vi "船舶健康监测7.22.vi"() -> ()   [LabVIEW 2018]
uses:
  D:/labview2018/LabVIEW 2018/examples/Connectivity/Python/support/PythonVersionsEnum.ctl
  <vilib>/Instr/_visa.llb/VISA Configure Serial Port (Instr).vi
  <vilib>/picture/3D Picture Control/Object/Add Object (no reference).vi
  <vilib>/picture/3D Picture Control/NI_3D Picture Control.lvlib
panel:
  in  "钉钉机器人开关":bool
  in  "Python版本":T1
  in  "VISA资源名称":refnum<visa-resource-name>
  out "?":refnum<vi>(3d-picture)
  out "?":refnum<vi>(3d-picture)
  out "?":refnum<vi>(3d-picture)
  out "?":i32(graph)
  out "?":i32(graph)
  out "?":i32(graph)
  out "?":i32(graph)
  out "?":i32(graph)
  in  "baud rate (9600)":u32=9600 caption="波特率"
  out "?":i32(graph)
  out "?":string
  out "下弯超过阈值":bool
  out "上弯超过阈值":bool
  out "原始数据":string
  in  "下阈值":dbl
  in  "上阈值":dbl
  in  "?":bool
  # "船舶健康监测数据显示平台"
  # "功能与使用说明：\n1.应变：实现实时图标显示应变值；阈值报警；周期内统计上传至onenet平台；钉钉机器人报警系统；保存至.txt格式文件。\n\n2.温湿度：实现实时图表显示；保存至.txt文件；\n\n3.姿态：实现实时图表显示；三维动态显示"
  # "应变"
  # "温度"
  # "Roll"
  # "湿度"
  # "Pitch"
  # "阈值\n报警"
  # "钉钉\n机器人"
  # "未开发"
  # "写入\n文件\n.txt"
  # "串口配置"
  # "Yallh"
  # "未开发"
  # "未开发"
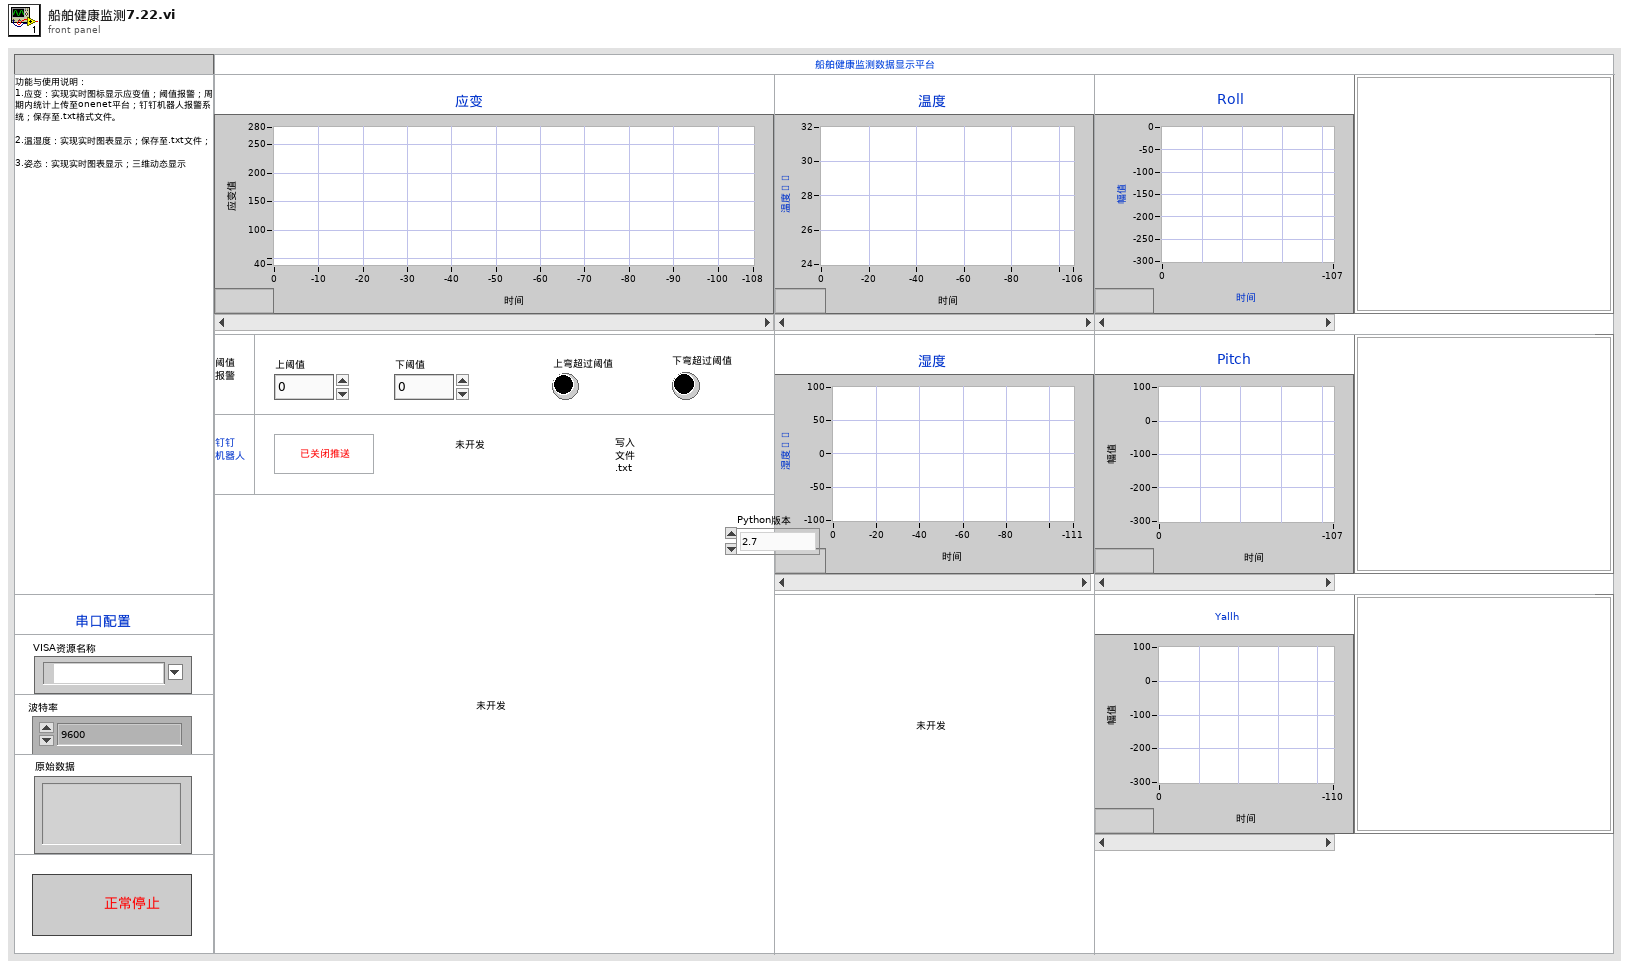
[diagram p1: front panel]
types:
  T1 = typedef "PythonVersionsEnum.ctl" = enum16{"2.7", "3.6"}
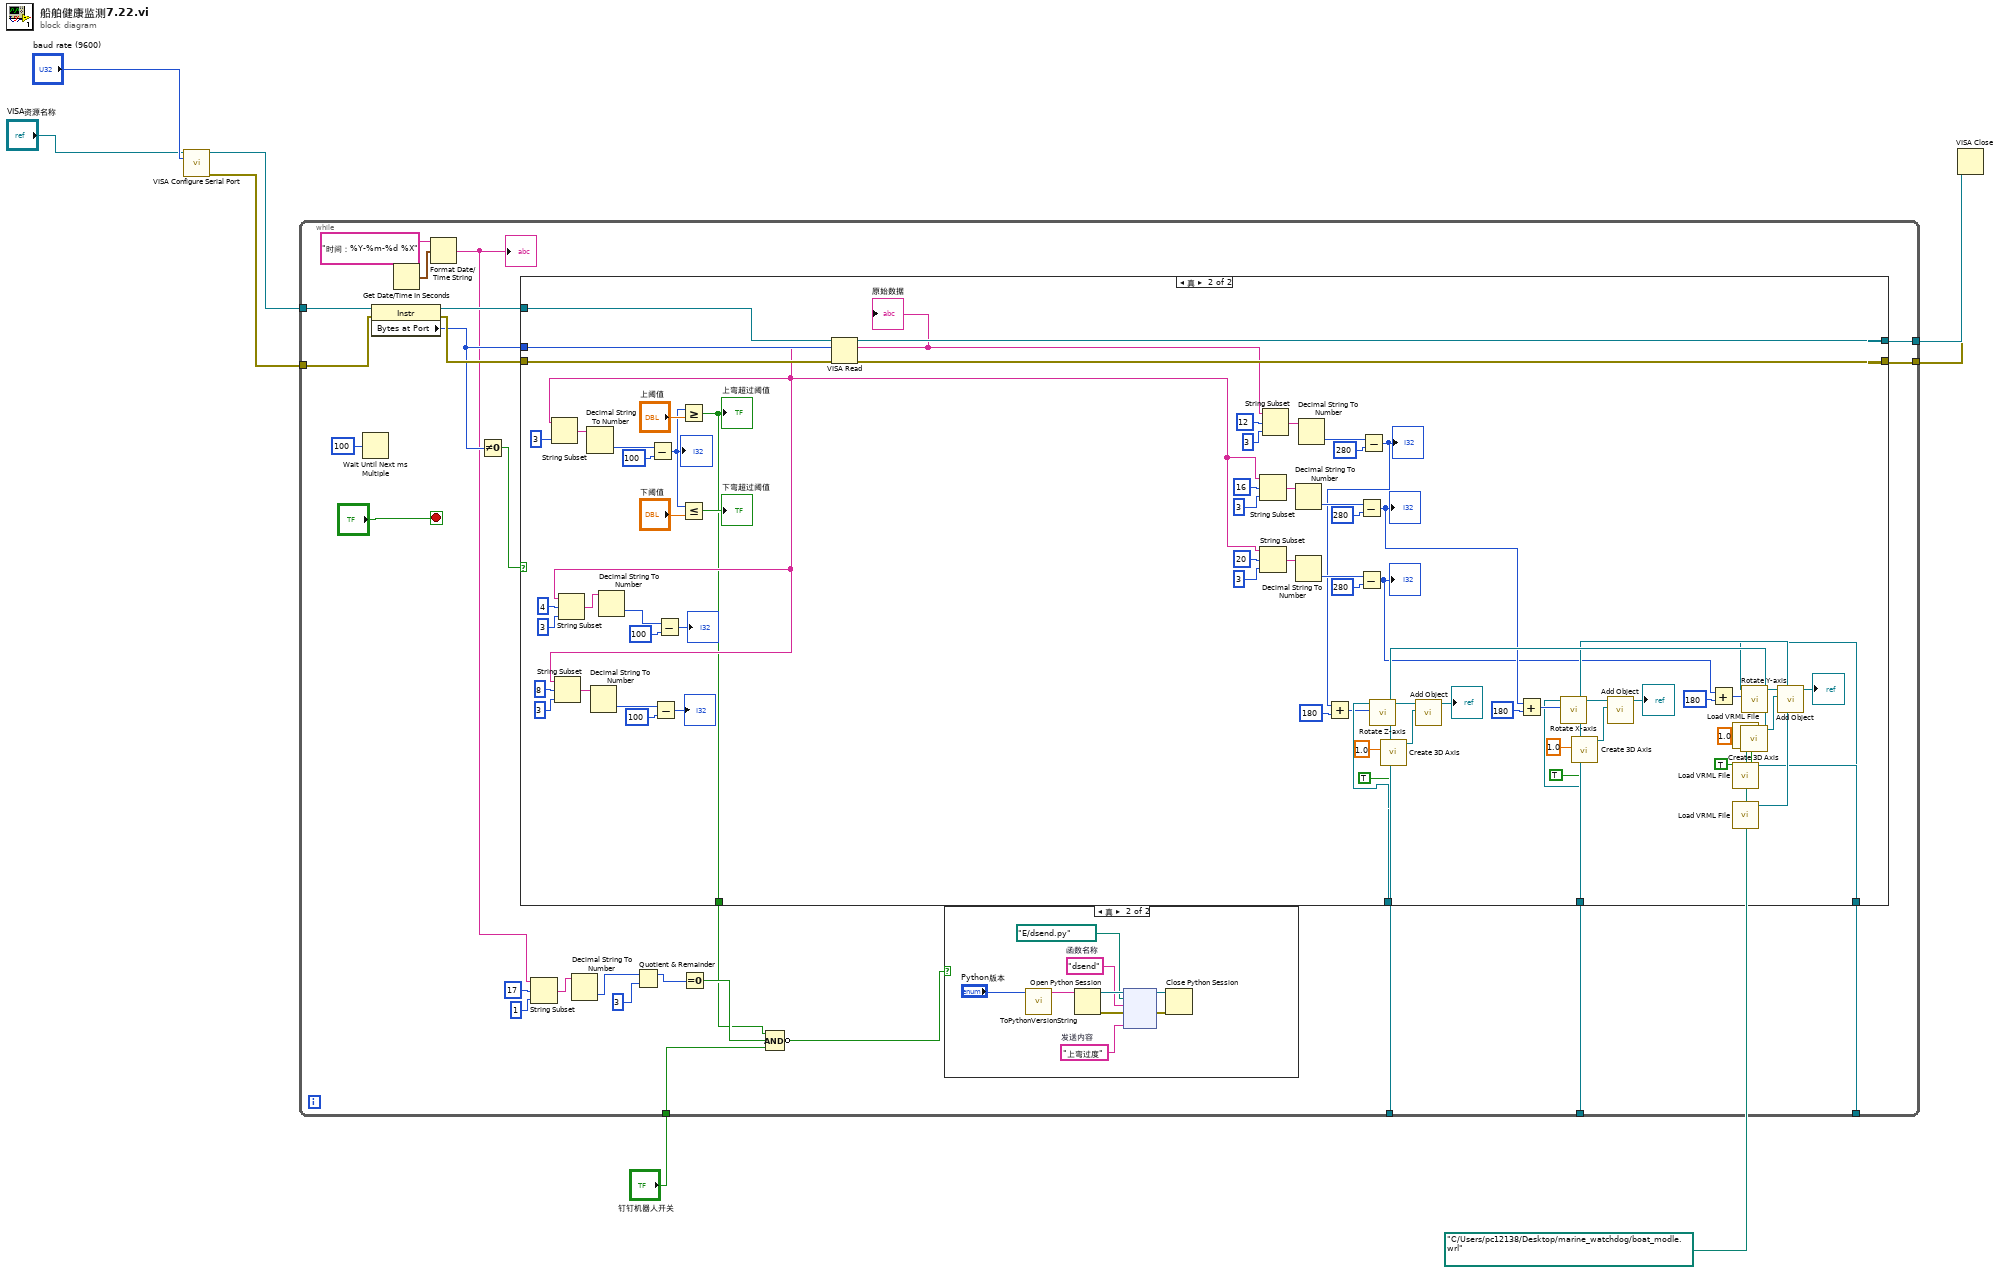
[diagram p0: block diagram]
diagram:
  w3 = path "C:/Users/pc12138/Desktop/marine_watchdog/boat_modle.wrl" ("Path")
  n1 = call-poly "VISA Configure Serial Port"("VISA resource name"="VISA资源名称", "baud rate (9600)"="baud rate (9600)") -> ("VISA resource name out"=w9:refnum<visa-resource-name>, "error out"=w8:errorcluster)  [unwired: 12 in]
  n2 = call <vilib>:"Load VRML File.vi"("Path"=w3) -> ("Scene:Read Scene File"=w6:refnum<vi>)  [unwired: 9 in, 1 out]
  n3 = call <vilib>:"Load VRML File.vi"("Path"=w3) -> ("Scene:Read Scene File"=w2:refnum<vi>)  [unwired: 9 in, 1 out]
  n4 = call <vilib>:"Load VRML File.vi"("Path"=w3) -> ("Scene:Read Scene File"=w5:refnum<vi>)  [unwired: 9 in, 1 out]
  n5 = while {
    tunnel: w8 -> [w37]
    tunnel: w9 -> [w34]
    tunnel: [w30] -> w11
    tunnel: [w29] -> w10
    tunnel: w6 -> [w25]
    tunnel: w5 -> [w24]
    tunnel: w2 -> [w23]
    tunnel: "钉钉机器人开关" -> [w15]
    stop <- "?" stop-if-true
    n6 = Wait Until Next ms Multiple(millisecond multiple=u32 100 ("毫秒倍数")) -> ()  [unwired: 1 out]
    n7 = property class="Instr"(reference=w34, error in=w37) -> (reference out=w35:refnum<visa-resource-name>, error out=w36:errorcluster, "Bytes at Port"=w33:u32)
    n8 = Get Date/Time In Seconds() -> (seconds since 1Jan1904=w28:timestamp)
    n9 = Format Date/Time String(time format string (%c)="时间：%Y-%m-%d %X", seconds (now)=w28) -> (date/time string=w19:string)  [unwired: 1 in]
    "?" <- w19
    n10 = Not Equal To 0?(x=w33) -> (x != 0?=w26:bool)
    n11 = case shown="真" w26 {
      tunnel: w36 -> [_ w115]
      tunnel: w35 -> [_ w114]
      tunnel: w33 -> [_ w113]
      tunnel: [_ w112] -> w30
      tunnel: [_ w111] -> w29
      tunnel: w25 -> [_ w74]
      tunnel: w24 -> [_ w51]
      tunnel: w23 -> [_ w48]
      tunnel: [_ w47] -> w13
      frame False {
      }
      frame True {
        n12 = VISA Read(VISA resource name=w114, byte count=w113, error in (no error)=w115) -> (VISA resource name out=w112:refnum<visa-resource-name>, read buffer=w75:string, error out=w111:errorcluster)  [unwired: 1 out]
        "原始数据" <- w75
        n13 = String Subset(string=w75, length (rest)=3 ("长度（剩余）")) -> (substring=w106:string)  [unwired: 1 in]
        n14 = String Subset(string=w75, offset (0)=8 ("偏移量(0)"), length (rest)=3 ("长度（剩余）")) -> (substring=w103:string)
        n15 = String Subset(string=w75, offset (0)=4 ("偏移量(0)"), length (rest)=3 ("长度（剩余）")) -> (substring=w102:string)
        n16 = Decimal String To Number(string=w106) -> (number=w99:i32)  [unwired: 2 in, 1 out]
        n17 = Decimal String To Number(string=w103) -> (number=w96:i32)  [unwired: 2 in, 1 out]
        n18 = Decimal String To Number(string=w102) -> (number=w93:i32)  [unwired: 2 in, 1 out]
        n19 = Subtract(x=w99, y=100) -> (x-y=w98:i32)
        "?" <- w98
        n20 = Subtract(x=w96, y=100) -> (x-y=→"?":i32)
        n21 = Subtract(x=w93, y=100) -> (x-y=→"?":i32)
        n22 = Greater Or Equal?(x=w98, y="上阈值") -> (x >= y?=w47:bool)
        "上弯超过阈值" <- w47
        n23 = Less Or Equal?(x=w98, y="下阈值") -> (x <= y?=→"下弯超过阈值":bool)
        n24 = String Subset(string=w75, offset (0)=16 ("偏移量(0)"), length (rest)=3 ("长度（剩余）")) -> (substring=w85:string)
        n25 = String Subset(string=w75, offset (0)=20 ("偏移量(0)"), length (rest)=3 ("长度（剩余）")) -> (substring=w76:string)
        n26 = String Subset(string=w75, offset (0)=12 ("偏移量(0)"), length (rest)=3 ("长度（剩余）")) -> (substring=w86:string)
        n27 = Decimal String To Number(string=w85) -> (number=w82:i32)  [unwired: 2 in, 1 out]
        n28 = Decimal String To Number(string=w76) -> (number=w79:i32)  [unwired: 2 in, 1 out]
        n29 = Decimal String To Number(string=w86) -> (number=w89:i32)  [unwired: 2 in, 1 out]
        n30 = Subtract(x=w82, y=280) -> (x-y=w50:i32)
        "?" <- w50
        n31 = Subtract(x=w79, y=280) -> (x-y=w49:i32)
        "?" <- w49
        n32 = Subtract(x=w89, y=280) -> (x-y=w68:i32)
        "?" <- w68
        n33 = Add(x=w68, y=180) -> (x+y=w67:i32)
        n34 = call <vilib>:"Rotate Z-axis.vi"("angle"=w67, "Scene Object In"=w74) -> ("Scene Object Out"=w71:refnum<vi>)  [unwired: 8 in, 1 out]
        n35 = call <vilib>:"Create 3D Axis.vi"("Axis label?"=TRUE, "Length"=sgl 1.0) -> ("New Object Refnum"=w70:refnum<vi>)  [unwired: 8 in, 1 out]
        n36 = call-poly <vilib>:"Add Object.vi"("New Object In"=w70, "Scene Object In"=w71) -> ("Scene Object Out"=→"?":refnum<vi>)  [unwired: 8 in, 1 out]
        n37 = Add(x=w50, y=180) -> (x+y=w64:i32)
        n38 = call <vilib>:"Rotate X-axis.vi"("angle"=w64, "Scene Object In"=w51) -> ("Scene Object Out"=w61:refnum<vi>)  [unwired: 8 in, 1 out]
        n39 = call <vilib>:"Create 3D Axis.vi"("Axis label?"=TRUE, "Length"=sgl 1.0) -> ("New Object Refnum"=w62:refnum<vi>)  [unwired: 8 in, 1 out]
        n40 = call-poly <vilib>:"Add Object.vi"("New Object In"=w62, "Scene Object In"=w61) -> ("Scene Object Out"=→"?":refnum<vi>)  [unwired: 8 in, 1 out]
        n41 = Add(x=w49, y=180) -> (x+y=w53:i32)
        n42 = call <vilib>:"Create 3D Axis.vi"("Axis label?"=TRUE, "Length"=sgl 1.0) -> ("New Object Refnum"=w55:refnum<vi>)  [unwired: 8 in, 1 out]
        n43 = call <vilib>:"Rotate Y-axis.vi"("angle"=w53, "Scene Object In"=w48) -> ("Scene Object Out"=w56:refnum<vi>)  [unwired: 8 in, 1 out]
        n44 = call-poly <vilib>:"Add Object.vi"("New Object In"=w55, "Scene Object In"=w56) -> ("Scene Object Out"=→"?":refnum<vi>)  [unwired: 8 in, 1 out]
      }
    }
    n45 = String Subset(string=w19, offset (0)=17 ("偏移量(0)"), length (rest)=1 ("长度（剩余）")) -> (substring=w20:string)
    n46 = Decimal String To Number(string=w20) -> (number=w18:i32)  [unwired: 2 in, 1 out]
    n47 = Quotient & Remainder(x=w18, y=3) -> (x-y*floor(x/y)=w16:i32)  [unwired: 1 out]
    n48 = Equal To 0?(x=w16) -> (x = 0?=w14:bool)
    n49 = Compound Arithmetic op=AND ("复合运算")(w13, w14, w15) -> (invert w12:bool)
    n50 = case shown="真" w12 {
      frame False {
      }
      frame True {
        w38 = "上弯过度"  # 发送内容
        w42 = "dsend"  # 函数名称
        n51 = call "ToPythonVersionString.vi"("Python版本"="Python版本") -> ("python版本字符串"=w46:string)  [unwired: 10 in]
        n52 = Open Python Session(python version=w46) -> (session out=w44:refnum<k35>, error out=w43:errorcluster)  [unwired: 2 in]
        n53 = node(w44, path "E:/dsend.py" ("模块路径"), w42, w43, w38) -> (w41:refnum<k35>, w40:errorcluster)  [unwired: 3 in, 2 out]
        n54 = Close Python Session(session in=w41, error in=w40) -> ()  [unwired: 1 out]
      }
    }
  }
  n55 = VISA Close(VISA resource name=w11, error in (no error)=w10) -> ()  [unwired: 1 out]
